vi "Analysis Plots.vi"(7 "action":T3, 8 "error in":errorcluster, 10 "challenge":T1={"compound"="toluene", "quantity"=0.0, "units"=enum."ppt", "comment"="BG1"}, 11 "IMS spectrum":dbl[](array[numeric])) -> (0 "error out":errorcluster, 2 "challenges":T1[](array[typedef]), 3 "plots":dbl[][](array[numeric]))   [LabVIEW 2011]
uses:
  Analysis Data.ctl
  Controls/Challenge.ctl
  Controls/Concentration Units.ctl
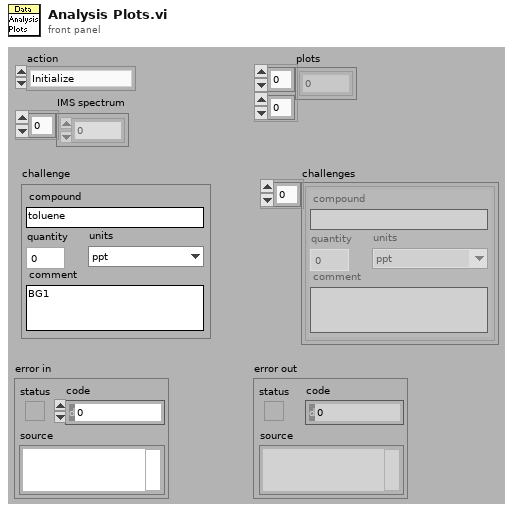
[diagram p1: front panel]
types:
  T1 = typedef "Challenge.ctl" = cluster{"compound":string, "quantity":dbl, "units":T2, "comment":string}
  T2 = typedef "Concentration Units.ctl" = enum16{"ppt", "ppb", "ppm"}
  T3 = typedef "Analysis Data.ctl" = enum16{"Initialize", "Add Plot", "Get Plots"}
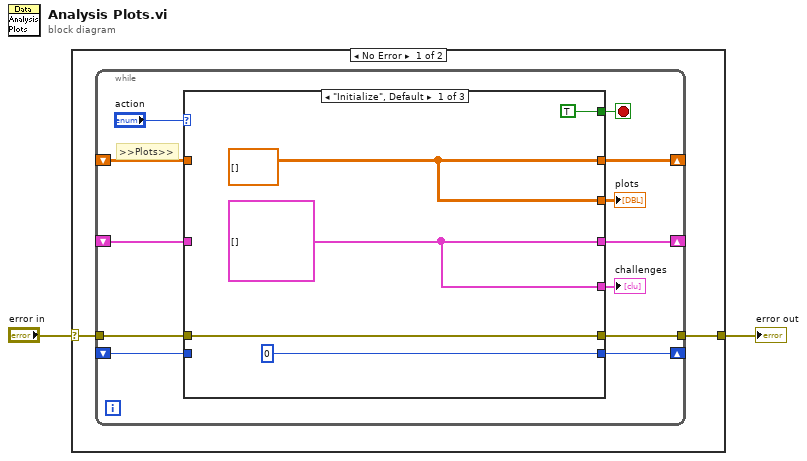
[diagram p0: block diagram]
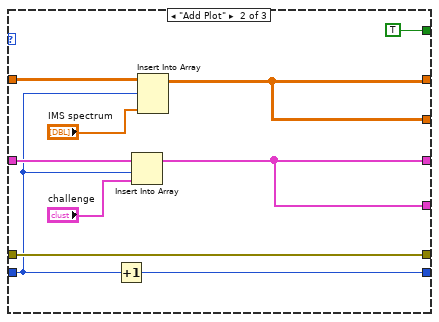
[diagram p2: hidden frame]
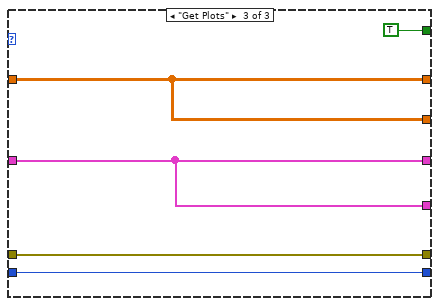
[diagram p3: hidden frame]
diagram:
  n1 = case shown="No Error" "error in" {
    selector: "error in" -> [w4 w37]
    tunnel: [w3 w37] -> w1
    frame No Error {
      n2 = while {
        shift-right: [w16] -> _
        shift-left: _ -> [w15]
        shift-right: [w14] -> _
        shift-left: _ -> [w13]
        tunnel: w4 -> [w12]
        tunnel: [w11] -> w3
        shift-right: [w6] -> _
        shift-left: _ -> [w7]
        stop <- w10 stop-if-true
        # ">>Plots>>"
        n3 = case shown="\"Initialize\", Default" "action" {
          tunnel: [w18 w26 w33] -> w16
          tunnel: w15 -> [_ w30 w33]
          tunnel: [0 w29 w34] -> w14
          tunnel: w13 -> [_ w23 w34]
          tunnel: w12 -> [w20 w28 w35]
          tunnel: [w20 w28 w35] -> w11
          tunnel: [TRUE TRUE TRUE] -> w10
          tunnel: [w18 w26 w33] -> w8
          tunnel: w7 -> [_ w25 w32]
          tunnel: [w17 w22 w32] -> w6
          tunnel: [w17 w22 w32] -> w5
          frame "Initialize", Default {
            w17 = T1[] []
            w18 = dbl[][] []
          }
          frame "Add Plot" {
            n4 = Increment(x=w23) -> (x+1=w29:i32)
            n5 = Insert Into Array(array=w25, index=w23, new element="challenge") -> (w22:T1[])
            n6 = Insert Into Array(array=w30, index (row)=w23, new element="IMS spectrum") -> (w26:dbl[][])  [unwired: 1 in]
          }
          frame "Get Plots" {
          }
        }
        "plots" <- w8
        "challenges" <- w5
      }
    }
    frame Error {
    }
  }
  "error out" <- w1
